vi "LowMasterFollower.vi"() -> ()   [LabVIEW 2019]
uses:
  Global Variables/Current K6221 Coarse.vi
  Global Variables/Voltage K24xx Coarse.vi
  Global Variables/Voltage K230 Coarse.vi
  Global Variables/Voltage Yokogawa Coarse.vi
panel:
  in  "Update Frequency (sec)":dbl=1.0 min=0.05 step=0.05
  in  "Monitor Stop":bool
  out "Voltage Yokogawa Coarse (V)":dbl
  out "Voltage K230 Coarse (V)":dbl
  out "Voltage K24xx Coarse (V)":dbl
  out "Current K6221 Coarse (A)":dbl
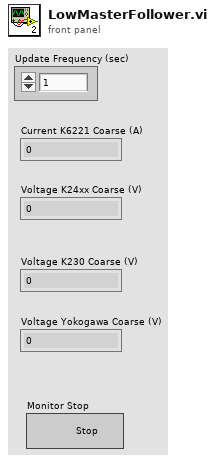
[diagram p1: front panel]
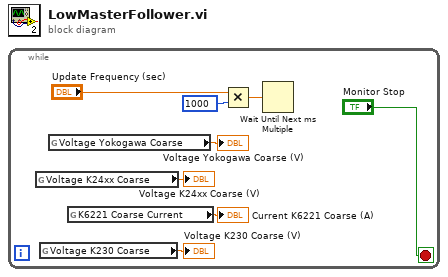
[diagram p0: block diagram]
diagram:
  n1 = while {
    stop <- "Monitor Stop" stop-if-true
    n2 = global read "Voltage K24xx Coarse.vi" "Voltage K24xx Coarse"() -> (→"Voltage K24xx Coarse (V)":dbl)
    n3 = global read "Voltage K230 Coarse.vi" "Voltage K230 Coarse"() -> (→"Voltage K230 Coarse (V)":dbl)
    n4 = global read "Voltage Yokogawa Coarse.vi" "Voltage Yokogawa Coarse"() -> (→"Voltage Yokogawa Coarse (V)":dbl)
    n5 = global read "Current K6221 Coarse.vi" "K6221 Coarse Current"() -> (→"Current K6221 Coarse (A)":dbl)
    n6 = Multiply(x="Update Frequency (sec)", y=u32 1000) -> (x*y=w6:dbl)
    n7 = Wait Until Next ms Multiple(millisecond multiple=w6) -> ()  [unwired: 1 out]
  }
